vi "VeriAlarma.vi"(2 "Temp Min":dbl, 3 "Temp Max":dbl, 4 "Nombre del archivo txt":string="Alarma.txt", 5 "Temp grados C":string="Temperatura baja", 7 "Grados C":dbl) -> (0 "Alarma":string, 1 "Notify Datos":T1)   [LabVIEW 2019]
doc: "Mediante la temperatura máxima y mínima adquirida esta es verificada (Guardar alertas o no) en un rango determinado por el usuario, para posteriormente ser guardada en un archivo de texto, con su respectiva estampa de tiempo y temperatura."
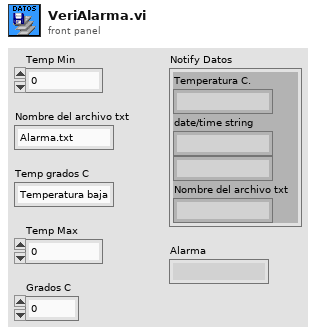
[diagram p1: front panel]
types:
  T1 = cluster{"Temperatura C.":string, "date/time string":string, string, "Nombre del archivo txt":string}
  T2 = cluster{"Temp grados C":string, "date/time string":string, string, "Nombre del archivo txt":string}
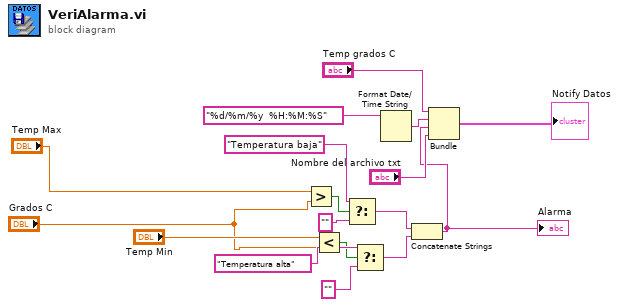
[diagram p0: block diagram]
diagram:
  n1 = Greater?(x="Temp Max", y="Grados C") -> (0:w3:bool)
  n2 = Less?(x="Temp Min", y="Grados C") -> (x < y?=w6:bool)
  n3 = Select(t="Temperatura baja" ("Nombre del archivo txt"), s=w3, f="" ("Nombre del archivo txt")) -> (s? t:f=w8:string)
  n4 = Select(t="Temperatura alta" ("Nombre del archivo txt"), s=w6, f="" ("Nombre del archivo txt")) -> (s? t:f=w9:string)
  n5 = Format Date/Time String(time format string (%c)="%d/%m/%y  %H:%M:%S") -> (date/time string=w2:string)  [unwired: 2 in]
  n6 = Concatenate Strings(w8, w9) -> (w10:string)
  "Alarma" <- w10
  n7 = Bundle("Temp grados C"="Temp grados C", "date/time string"=w2, w10, "Nombre del archivo txt"="Nombre del archivo txt") -> (→"Notify Datos":T2)  [unwired: 1 in]
